vi "Read Version.vi"(8 "error in (no error)":errorcluster, 11 "Engine Simulation IP in":refnum<class "Engine Simulation IP.lvclass">) -> (0 "error out":errorcluster, 2 "version":T1, 3 "Engine Simulation IP out":refnum<class "Engine Simulation IP.lvclass">)   [LabVIEW 2013, in "Engine Simulation IP.lvclass"]
uses:
  Engine Simulation IP.lvclass
  Bitfile Major Version.ctl
  Engine Simulation IP.lvclass/Engine Simulation IP.ctl
  Engine Simulation Session.lvclass
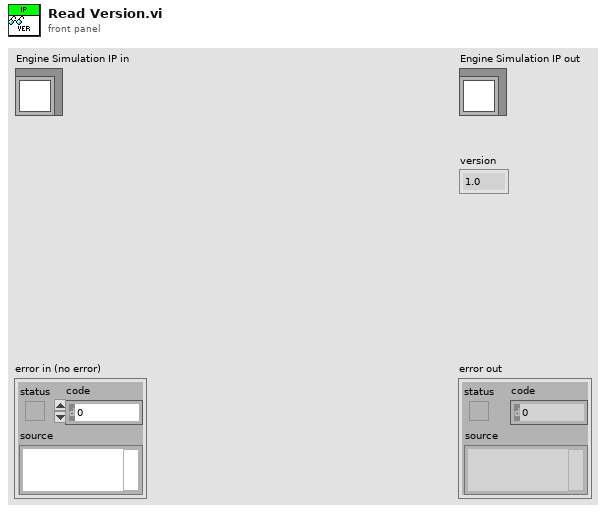
[diagram p1: front panel]
types:
  T1 = typedef "Engine Simulation Session.lvclass/Bitfile Major Version.ctl" = enum16{"1.0", "1.1", "1.2", "1.3"}
  T2 = typedef "Engine Simulation IP.lvclass/IP class private data.ctl" = cluster{"Name":string, "EST version":T1, "session":refnum<class "Engine Simulation Session.lvclass">}
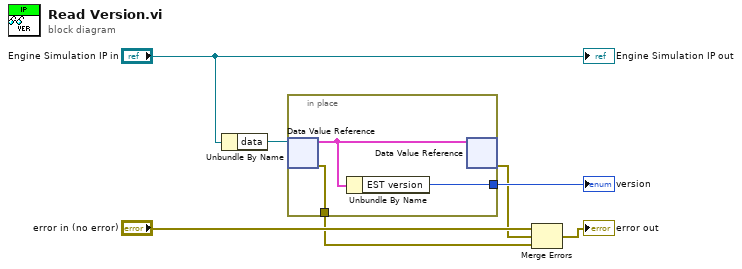
[diagram p0: block diagram]
diagram:
  n1 = Unbundle By Name("Engine Simulation IP in") -> ("data"=w5:refnum<data-value>)
  n2 = in-place {
    in-place-border: [w9] -> w4
    in-place-border: [w8] -> w2
    n3 = in-place-dvr #1(w5) -> (w10:T2, w8:errorcluster)
    n4 = Unbundle By Name(w10) -> ("EST version"=w9:T1)
    n5 = in-place-dvr #1(w10) -> (w1:errorcluster)  [unwired: 1 out]
  }
  "version" <- w4
  n6 = Merge Errors("error in (no error)", w1, w2) -> (→"error out":errorcluster)
  "Engine Simulation IP out" <- "Engine Simulation IP in"
